vi "Actor Core.vi"(8 "error in":errorcluster, 11 "Data Logger Display in":refnum<class "Data Logger Display.lvclass">) -> (0 "error out":errorcluster, 3 "Actor out":refnum<class "Actor.lvclass">)   [LabVIEW 2013, in "Display Panel.lvlib" / "Data Logger Display.lvclass"]
doc: "(<B>Filename</B>: Actor Framework.lvlib:Actor.lvclass:Actor Core.vi)\n\nReceives messages to the actor, reacts to them, and initiates any error handling that may shut the actor down.\n\nDescendant classes may override this VI to append parallel tasks for the actor to complete while it handles messages. Overrides use the Call Parent Method node."
uses:
  Data Logger Display.lvclass
  <vilib>/ActorFramework/Actor/Actor.lvclass
  Abstract Display/Abstract Display.lvclass/Abstract Display.ctl
  Abstract Display/Abstract Display.lvclass
  <vilib>/ActorFramework/Message Enqueuer/Init from Existing Queue.vi
  <vilib>/ActorFramework/Message Enqueuer/Message Enqueuer.lvclass
panel:
  out "Blinker":bool
  in  "Exit":bool
  in  "Stop":bool
  out "Card #":dbl
  out "Time":dbl format="%<%H:%M:%S>t"
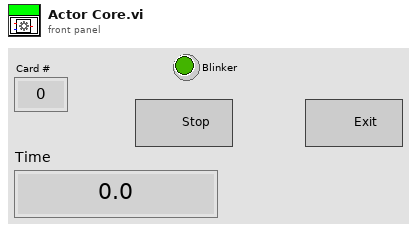
[diagram p1: front panel]
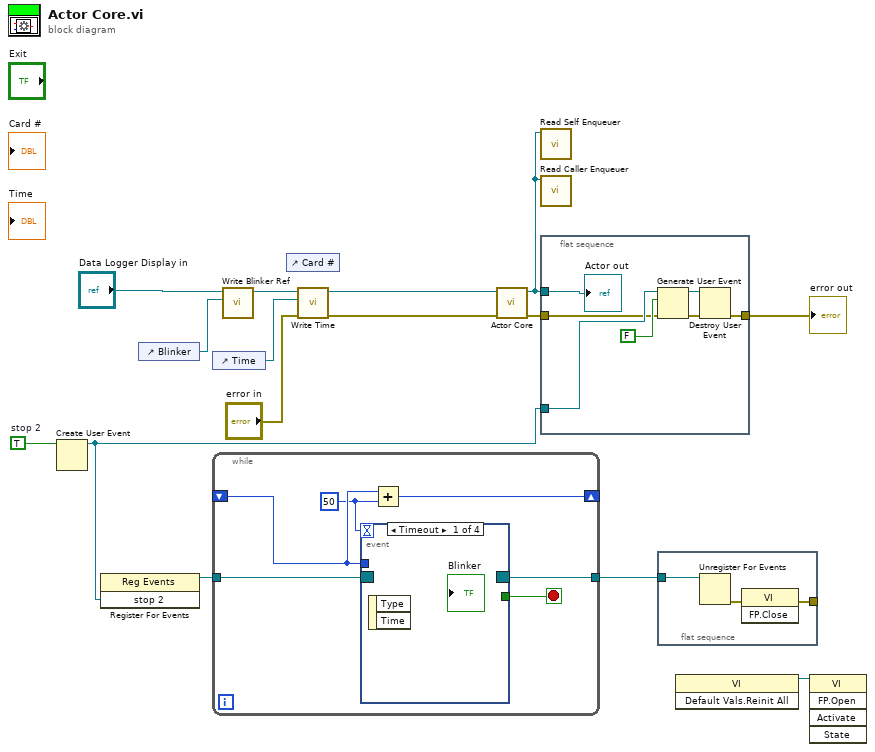
[diagram p0: block diagram]
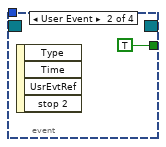
[diagram p2: hidden frame]
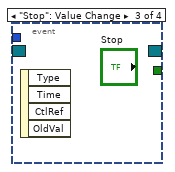
[diagram p3: hidden frame]
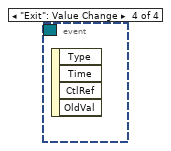
[diagram p4: hidden frame]
diagram:
  w14 = TRUE  # stop 2
  n1 = Create User Event(user event datatype=w14) -> (user event=w13:refnum<user-event>)  [unwired: 1 in, 1 out]
  n2 = register-events(w13) -> (reference out=w11:refnum<event-registration>)  [unwired: 2 in, 1 out]
  n3 = control-ref of="Blinker"() -> (w3:refnum<vi>)
  n4 = control-ref of="Time"() -> (w7:refnum<vi>)
  n5 = while {
    tunnel: w11 -> [w21]
    tunnel: [w20] -> w10
    shift-right: [w17] -> _
    shift-left: _ -> [w19]
    stop <- w16 stop-if-true
    w18 = 50
    n6 = event shown="[0] Timeout" {
      selector: w21 -> [_ _ _ _]
      dyn-events: [_ _ _ _] -> w20
      timeout: w18 -> [_ _ _ _]
      tunnel: w19 -> [_ _ _ _]
      tunnel: [_ TRUE _ _] -> w16
      event Timeout {
        n7 = event-data() -> ()  [unwired: 1 in, 2 out]
      }
      event User Event {
        n8 = event-data() -> ()  [unwired: 1 in, 4 out]
      }
      event "Stop": Value Change {
        n9 = event-data() -> ()  [unwired: 1 in, 4 out]
      }
      event "Exit": Value Change {
        n10 = event-data() -> ()  [unwired: 1 in, 4 out]
      }
    }
    n11 = Add(x=w19, y=w18) -> (x+y=w17:i32)
  }
  n12 = call "Write Blinker Ref.vi"("Blinker Ref"=w3, "Abstract Display in"="Data Logger Display in") -> ("Abstract Display out"=w4:refnum<class "Data Logger Display.lvclass">)  [unwired: 8 in, 1 out]
  n13 = control-ref of="Card #"() -> ()  [unwired: 1 out]
  n14 = call "Write Time.vi"("error in (no error)"="error in", "Time"=w7, "Abstract Display in"=w4) -> ("error out"=w1:errorcluster, "Abstract Display out"=w2:refnum<class "Data Logger Display.lvclass">)  [unwired: 7 in]
  n15 = call-parent "Actor Core.vi"("error in"=w1, "Abstract Display in"=w2) -> ("error out"=w15:errorcluster, "Actor out"=w8:refnum<class "Actor.lvclass">)  [unwired: 8 in]
  n16 = call <vilib>:"Read Self Enqueuer.vi"("Actor"=w8) -> ()  [unwired: 10 in, 1 out]
  n17 = call <vilib>:"Read Caller Enqueuer.vi"("Actor"=w8) -> ()  [unwired: 10 in, 1 out]
  n18 = flat-sequence {
    tunnel: w15 -> [w25]
    tunnel: w8 -> [w29]
    tunnel: w13 -> [w26]
    tunnel: [w23] -> w12
    frame #0 {
      n19 = Generate User Event(user event=w26, event data cluster=FALSE ("event data"), error in=w25) -> (user event out=w28:refnum<user-event>, error out=w24:errorcluster)  [unwired: 1 in]
      n20 = Destroy User Event(user event=w28, error in=w24) -> (error out=w23:errorcluster)
      "Actor out" <- w29
    }
  }
  n21 = flat-sequence {
    tunnel: w10 -> [w32]
    tunnel: [w30] -> _
    frame #0 {
      n22 = Unregister For Events(event registration refnum=w32) -> (error out=w31:errorcluster)  [unwired: 1 in]
      n23 = invoke class="VI" method="FP.Close"(error in=w31) -> (error out=w30:errorcluster)  [unwired: 2 in, 2 out]
    }
  }
  n24 = invoke class="VI" method="Default Vals.Reinit All"() -> (reference out=w9:refnum<vi>)  [unwired: 3 in, 2 out]
  n25 = invoke class="VI" method="FP.Open"(reference=w9) -> ()  [unwired: 4 in, 5 out]
  "error out" <- w12
